vi "Get Stream Samples Ready.vi"(8 "error in (no error)":errorcluster, 10 "stream index":i32, 11 "refnum in":refnum<k20>) -> (0 "error out":errorcluster, 2 "samples ready":u32, 3 "refnum out":refnum<k20>)   [LabVIEW 2015, in "niInstr Streaming v1 Host.lvlib"]
doc: "This coordinates with the FPGA-side stream VI - Monitor FIFO Health.vi. Specifically the FPGA client code should report the number of samples ready for consumption here. This is an optional interface, and is primarily useful for output DMA use-cases where priming a DMA FIFO is useful to ensure gapless transfer.\n\n<B>Input Parameters</B>\n\n<B>error in (no error)</B> 'error in' can accept error information wired from VIs previously called. Use this information to decide if any functionality should be bypassed in the event of errors from other VIs.\n\nRight-click the 'error in' control on the front panel and select 'Explain Error' or 'Explain Warning' from the shortcut menu for more information about the error.\n\n<B>stream index</B> Selects which stream index this VI will interface to. This is the index number at the end of the host interface controls (0..7).\n\n<B>refnum in</B> Wire in the session obtained from Open FPGA Reference.\n\n<B>Output Parameters</B>\n\n<B>error out</B> contains error information. This output provides standard error out functionality.\n\n<B>refnum out</B> Copy of refnum in"
uses:
  <instrlib>/_niInstr/Streaming/v1/Host/niInstr Streaming v1 Host.lvlib
  <instrlib>/_niInstr/Streaming/v1/Host/Public/Stream Host Interface.ctl
  <vilib>/Utility/error.llb/Error Cluster From Error Code.vi
  <vilib>/rvi/errors/niLvFpgaAdjustHostInterfaceError.vi
  <vilib>/ErrorRing/Error Ring.xnode
  <vilib>/rvi/interface/nirviReadWriteControl/nirviReadWriteControl.xnode
  <vilib>/rvi/interface/Simulation/niFpgaSimulationCallBeginRW.vi
  NiFpgaLv.dll
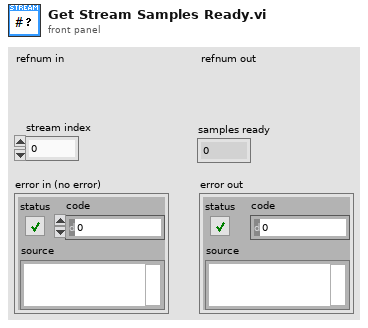
[diagram p1: front panel]
types:
  T1 = typedef "niInstr Streaming v1 Host.lvlib/Stream Host Interface.ctl" = refnum<k20>
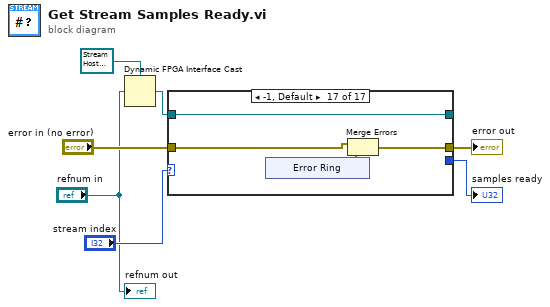
[diagram p0: block diagram]
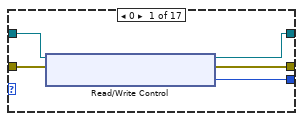
[diagram p2: hidden frame]
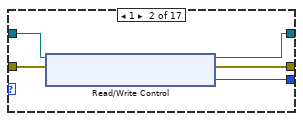
[diagram p3: hidden frame]
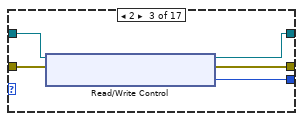
[diagram p4: hidden frame]
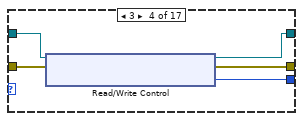
[diagram p5: hidden frame]
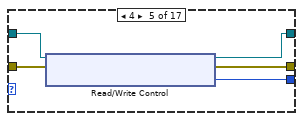
[diagram p6: hidden frame]
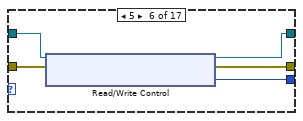
[diagram p7: hidden frame]
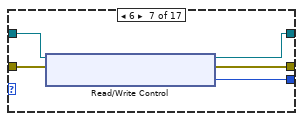
[diagram p8: hidden frame]
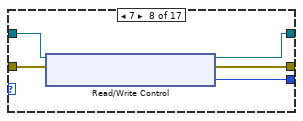
[diagram p9: hidden frame]
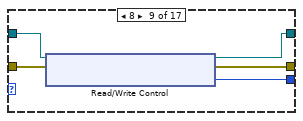
[diagram p10: hidden frame]
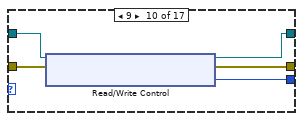
[diagram p11: hidden frame]
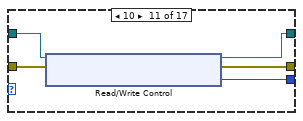
[diagram p12: hidden frame]
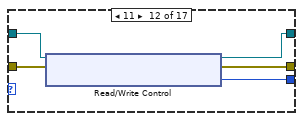
[diagram p13: hidden frame]
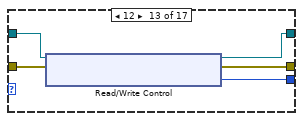
[diagram p14: hidden frame]
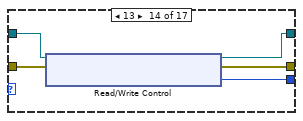
[diagram p15: hidden frame]
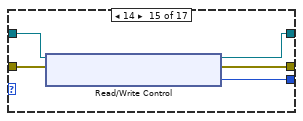
[diagram p16: hidden frame]
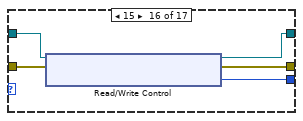
[diagram p17: hidden frame]
diagram:
  n1 = Dynamic FPGA Interface Cast(Session In=T1 refnum ("Refnum in"), Type="refnum in") -> (Session Out=w1:T1)
  n2 = case shown="-1, Default" "stream index" {
    tunnel: "error in (no error)" -> [w12 w17 w22 w27 w32 w37 w42 w47 w52 w57 w62 w67 w72 w77 w82 w87 w88]
    tunnel: [w11 w16 w21 w26 w31 w36 w41 w46 w51 w56 w61 w66 w71 w76 w81 w86 w91] -> _
    tunnel: [w10 w15 w20 w25 w30 w35 w40 w45 w50 w55 w60 w65 w70 w75 w80 w85 w89] -> w5
    tunnel: w1 -> [w9 w14 w19 w24 w29 w34 w39 w44 w49 w54 w59 w64 w69 w74 w79 w84 w91]
    tunnel: [w8 w13 w18 w23 w28 w33 w38 w43 w48 w53 w58 w63 w68 w73 w78 w83 _] -> w7
    frame 0 {
      n3 = xnode "Read/Write Control"("FPGA VI Reference In"=w9, "error in"=w12) -> ("FPGA VI Reference Out"=w11:T1, "error out"=w10:errorcluster, "stream.num samples ready 0"=w8:u32)
    }
    frame 1 {
      n4 = xnode "Read/Write Control"("FPGA VI Reference In"=w14, "error in"=w17) -> ("FPGA VI Reference Out"=w16:T1, "error out"=w15:errorcluster, "stream.num samples ready 1"=w13:u32)
    }
    frame 2 {
      n5 = xnode "Read/Write Control"("FPGA VI Reference In"=w19, "error in"=w22) -> ("FPGA VI Reference Out"=w21:T1, "error out"=w20:errorcluster, "stream.num samples ready 2"=w18:u32)
    }
    frame 3 {
      n6 = xnode "Read/Write Control"("FPGA VI Reference In"=w24, "error in"=w27) -> ("FPGA VI Reference Out"=w26:T1, "error out"=w25:errorcluster, "stream.num samples ready 3"=w23:u32)
    }
    frame 4 {
      n7 = xnode "Read/Write Control"("FPGA VI Reference In"=w29, "error in"=w32) -> ("FPGA VI Reference Out"=w31:T1, "error out"=w30:errorcluster, "stream.num samples ready 4"=w28:u32)
    }
    frame 5 {
      n8 = xnode "Read/Write Control"("FPGA VI Reference In"=w34, "error in"=w37) -> ("FPGA VI Reference Out"=w36:T1, "error out"=w35:errorcluster, "stream.num samples ready 5"=w33:u32)
    }
    frame 6 {
      n9 = xnode "Read/Write Control"("FPGA VI Reference In"=w39, "error in"=w42) -> ("FPGA VI Reference Out"=w41:T1, "error out"=w40:errorcluster, "stream.num samples ready 6"=w38:u32)
    }
    frame 7 {
      n10 = xnode "Read/Write Control"("FPGA VI Reference In"=w44, "error in"=w47) -> ("FPGA VI Reference Out"=w46:T1, "error out"=w45:errorcluster, "stream.num samples ready 7"=w43:u32)
    }
    frame 8 {
      n11 = xnode "Read/Write Control"("FPGA VI Reference In"=w49, "error in"=w52) -> ("FPGA VI Reference Out"=w51:T1, "error out"=w50:errorcluster, "stream.num samples ready 8"=w48:u32)
    }
    frame 9 {
      n12 = xnode "Read/Write Control"("FPGA VI Reference In"=w54, "error in"=w57) -> ("FPGA VI Reference Out"=w56:T1, "error out"=w55:errorcluster, "stream.num samples ready 9"=w53:u32)
    }
    frame 10 {
      n13 = xnode "Read/Write Control"("FPGA VI Reference In"=w59, "error in"=w62) -> ("FPGA VI Reference Out"=w61:T1, "error out"=w60:errorcluster, "stream.num samples ready 10"=w58:u32)
    }
    frame 11 {
      n14 = xnode "Read/Write Control"("FPGA VI Reference In"=w64, "error in"=w67) -> ("FPGA VI Reference Out"=w66:T1, "error out"=w65:errorcluster, "stream.num samples ready 11"=w63:u32)
    }
    frame 12 {
      n15 = xnode "Read/Write Control"("FPGA VI Reference In"=w69, "error in"=w72) -> ("FPGA VI Reference Out"=w71:T1, "error out"=w70:errorcluster, "stream.num samples ready 12"=w68:u32)
    }
    frame 13 {
      n16 = xnode "Read/Write Control"("FPGA VI Reference In"=w74, "error in"=w77) -> ("FPGA VI Reference Out"=w76:T1, "error out"=w75:errorcluster, "stream.num samples ready 13"=w73:u32)
    }
    frame 14 {
      n17 = xnode "Read/Write Control"("FPGA VI Reference In"=w79, "error in"=w82) -> ("FPGA VI Reference Out"=w81:T1, "error out"=w80:errorcluster, "stream.num samples ready 14"=w78:u32)
    }
    frame 15 {
      n18 = xnode "Read/Write Control"("FPGA VI Reference In"=w84, "error in"=w87) -> ("FPGA VI Reference Out"=w86:T1, "error out"=w85:errorcluster, "stream.num samples ready 15"=w83:u32)
    }
    frame -1, Default {
      n19 = xnode "Error Ring"() -> ("error out"=w90:errorcluster)
      n20 = Merge Errors(w88, w90) -> (w89:errorcluster)
    }
  }
  "samples ready" <- w7
  "error out" <- w5
  "refnum out" <- "refnum in"
